vi "DELETE Format DAQ Configuration Log.vi"(6 "Sweeping?":bool, 8 "error in (no error)":errorcluster, 10 "waveform":waveform(dbl)[](array[waveform]), 11 "Instrument.Lockin in":refnum<class "Instrument.Lockin.lvclass">) -> (0 "error out":errorcluster, 1 "Log Data":T1[](array[typedef]), 2 "Log Paths":string, 3 "Instrument.Lockin out":refnum<class "Instrument.Lockin.lvclass">, 4 "Times":timestamp[](array[timestamp]))   [LabVIEW 2019]
uses:
  Typedefs/Lockin.LogSweepAOAI--Cluster.ctl
  Instrument.Lockin.lvclass
  Instrument.Lockin.lvclass/Instrument.Lockin.ctl
  Instrument.DAQ/Instrument.DAQ.lvclass
  C:/Program Files/National Instruments/LabVIEW 2019/user.lib/LevyLab/Instrument Framework/Instrument Types/Lockin/Instrument.LockinAPI.lvclass
  C:/Program Files/National Instruments/LabVIEW 2019/user.lib/LevyLab/Instrument Framework/Instrument/Instrument.lvclass
  C:/Program Files/National Instruments/LabVIEW 2019/vi.lib/JKI/JKI SMO/SMO/SMO.lvclass
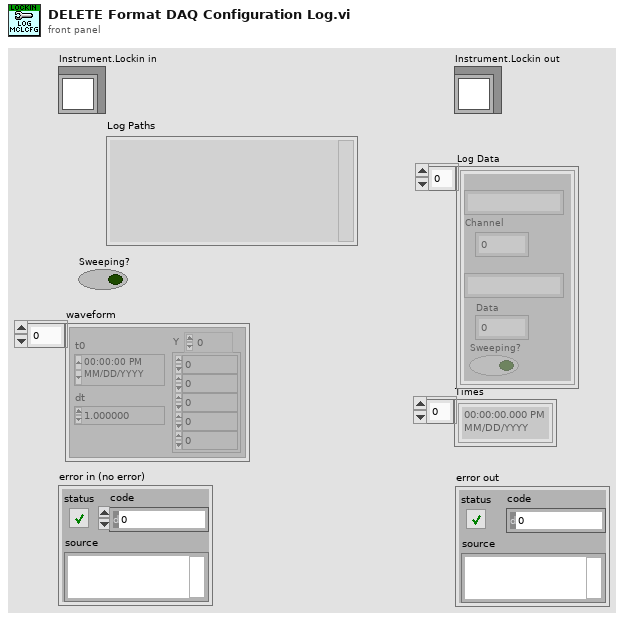
[diagram p1: front panel]
types:
  T1 = typedef "Instrument.Lockin.lvlib/Instrument.Lockin.lvclass/Lockin.LogSweepAOAI--Cluster.ctl" = cluster{"SystemSerialNumber":string, "Channel":i32, "Channel Type":string, "Data":dbl, "Sweeping?":bool}
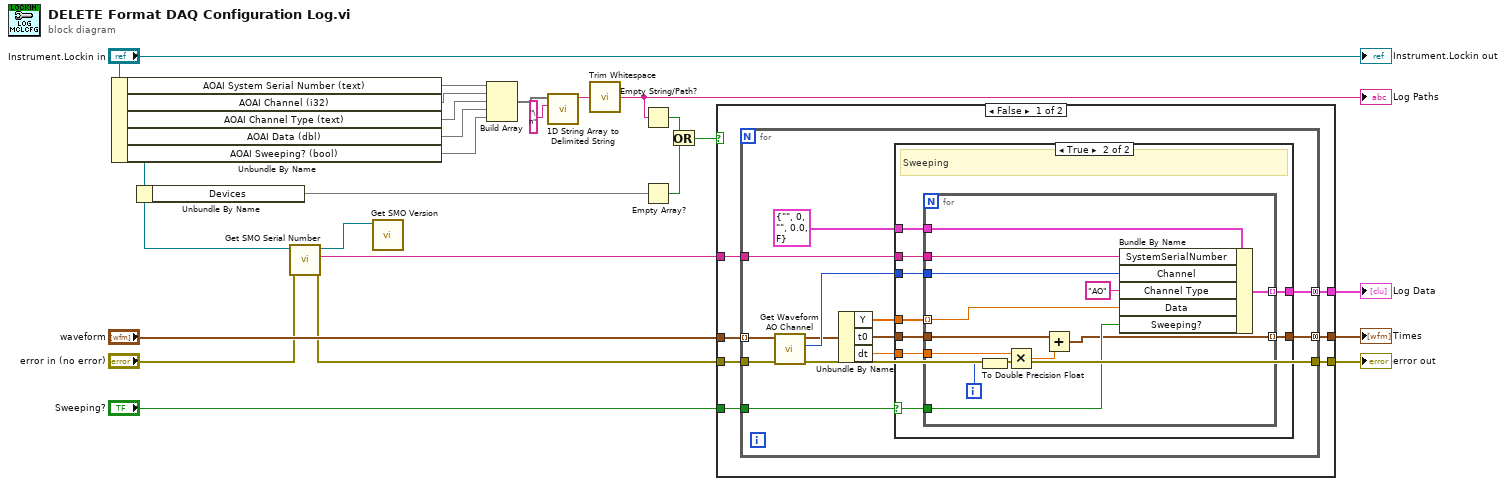
[diagram p0: block diagram]
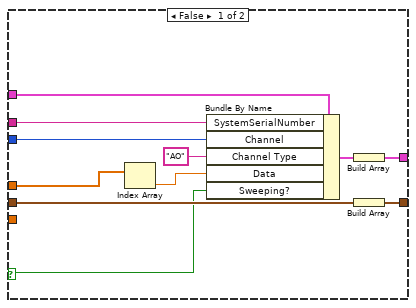
[diagram p2: hidden frame]
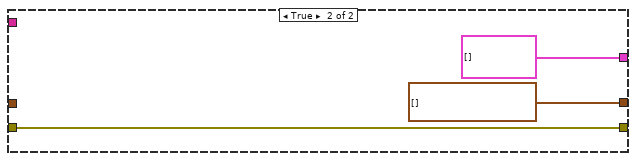
[diagram p3: hidden frame]
diagram:
  n1 = Unbundle By Name("Instrument.Lockin in") -> ("AOAI System Serial Number (text)"=w19, "AOAI Channel (i32)"=w6, "AOAI Channel Type (text)"=w5, "AOAI Data (dbl)"=w4, "AOAI Sweeping? (bool)"=w3)
  n2 = Unbundle By Name("Instrument.Lockin in") -> ("Devices"=w7)
  n3 = call-dynamic "Get SMO Serial Number.vi"("error in (no error)"="error in (no error)", "Instrument.Lockin in"="Instrument.Lockin in") -> ("error out"=w8:errorcluster, "Serial Number"=w10:string, "Instrument.Lockin out"=w1:refnum<class "Instrument.Lockin.lvclass">)  [unwired: 7 in]
  n4 = call-dynamic "Get SMO Version.vi"("Instrument.Lockin in"=w1) -> ()  [unwired: 8 in, 3 out]
  n5 = Build Array(w19, w6, w5, w4, w3) -> (w18:void[])
  n6 = call <vilib>:"1D String Array to Delimited String.vi"("delimiter"="\n", "string array"=w18) -> ("delimited string"=w12:string)  [unwired: 9 in]
  n7 = call <vilib>:"Trim Whitespace.vi"("string"=w12) -> ("trimmed string"=w11:string)  [unwired: 1 in]
  "Log Paths" <- w11
  n8 = Empty String/Path?(string/path=w11) -> (empty?=w14:bool)
  n9 = Empty Array?(array=w7) -> (empty?=w15:bool)
  n10 = Or(x=w14, y=w15) -> (x .or. y?=w13:bool)
  n11 = case shown="False" w13 {
    tunnel: [w30 timestamp[] []] -> w23
    tunnel: [w29 T1[] []] -> w22
    tunnel: "waveform" -> [w28 _]
    tunnel: "Sweeping?" -> [w27 _]
    tunnel: w8 -> [w26 w77]
    tunnel: w10 -> [w25 _]
    tunnel: [w24 w77] -> w16
    frame False {
      n12 = for {
        tunnel: [w43] -> w30 mode=concatenating
        tunnel: [w42] -> w29 mode=concatenating
        tunnel: w25 -> [w41]
        tunnel: w28 -> [w34] mode=indexing
        tunnel: w27 -> [w37]
        tunnel: w26 -> [w32]
        tunnel: [w31] -> w24
        n13 = call "Get Waveform AO Channel.vi"("error in (no error)"=w32, "Reference in"=w34) -> ("error out"=w31:errorcluster, "AO Channel"=w36:i32, "Reference out"=w35:waveform(dbl))  [unwired: 7 in]
        n14 = Unbundle By Name(w35) -> ("Y"=w40:dbl[], "t0"=w38:timestamp, "dt"=w39:dbl)
        n15 = case shown="True" w37 {
          selector: w37 -> [w45 w57]
          tunnel: [w50 w63] -> w43
          tunnel: [w52 w62] -> w42
          tunnel: w41 -> [w51 w61]
          tunnel: w40 -> [w47 w60]
          tunnel: w39 -> [_ w59]
          tunnel: w38 -> [w49 w58]
          tunnel: w36 -> [w48 w56]
          tunnel: T1 {"SystemSerialNumber"="", "Channel"=0, "Channel Type"="", "Data"=0.0, "Sweeping?"=FALSE} ("cluster") -> [w54 w55]
          frame False {
            n16 = Index Array(array=w47) -> (element=w46:dbl)  [unwired: 1 in]
            n17 = Bundle By Name(cluster=w54, "SystemSerialNumber"=w51, "Channel"=w48, "Channel Type"="AO", "Data"=w46, "Sweeping?"=w45) -> (w53:T1)
            n18 = Build Array(w53) -> (w52:T1[])
            n19 = Build Array(w49) -> (w50:timestamp[])
          }
          frame True {
            # "Sweeping"
            n20 = for {
              tunnel: w58 -> [w72]
              tunnel: w59 -> [w76]
              tunnel: [w64] -> w63 mode=indexing
              tunnel: w60 -> [w71] mode=indexing
              tunnel: w61 -> [w70]
              tunnel: w56 -> [w69]
              tunnel: w57 -> [w68]
              tunnel: [w67] -> w62 mode=indexing
              tunnel: w55 -> [w66]
              i -> [w75]
              n21 = To Double Precision Float(number=w75) -> (double precision float=w74:dbl)
              n22 = Multiply(x=w76, y=w74) -> (x*y=w73:dbl)
              n23 = Add(x=w72, y=w73) -> (x+y=w64:timestamp)
              n24 = Bundle By Name(cluster=w66, "SystemSerialNumber"=w70, "Channel"=w69, "Channel Type"="AO", "Data"=w71, "Sweeping?"=w68) -> (w67:T1)
            }
          }
        }
      }
    }
    frame True {
    }
  }
  "Times" <- w23
  "Log Data" <- w22
  "error out" <- w16
  "Instrument.Lockin out" <- "Instrument.Lockin in"
